vi "Upgrade to Secure Client VISA Socket.vi"(6 "server certificate validation":enum32{"Any Trusted CA", "None"}(ring), 7 "immutable TLS Configuration":refnum<k36>, 8 "error in (no error)":errorcluster, 9 "timeout (5000ms)":i32=5000, 10 "Server Hostname":string, 11 "VISA TCP Socket in":refnum<class "VISA TCP.lvclass">) -> (0 "error out":errorcluster, 2 "server certificate chain":cluster{"certificate":u8[]}[](array[cluster]), 3 "Secure VISA TCP Socket out":refnum<class "VISA TCP.lvclass">)   [LabVIEW 2020, in "Secure Sockets Addon.lvlib"]
doc: "Upgrades a Client VISA TCP socket to use SSL/TLS."
uses:
  <vilib>/MediaMongrels Ltd/WebSockets/Sockets/VISA TCP Socket/VISA TCP.lvclass
  <vilib>/MediaMongrels Ltd/WebSockets/Sockets/VISA TCP Socket/VISA TCP.lvclass/VISA TCP.ctl
  <vilib>/MediaMongrels Ltd/WebSockets/Sockets/VISA TCP Socket/Read TCP Refnum.vi
  <vilib>/MediaMongrels Ltd/WebSockets/Sockets/VISA TCP Socket/Write TCP Refnum.vi
  Secure Sockets Addon.lvlib
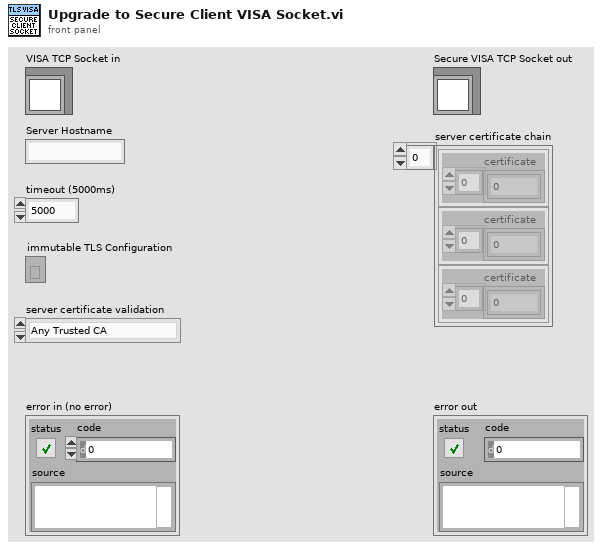
[diagram p1: front panel]
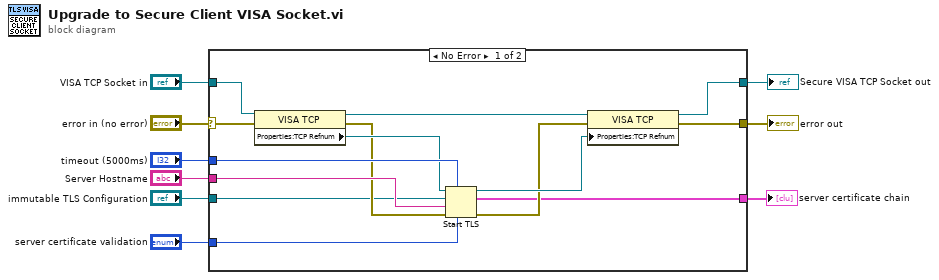
[diagram p0: block diagram]
diagram:
  n1 = case shown="No Error" "error in (no error)" {
    selector: "error in (no error)" -> [w13 w25]
    tunnel: "VISA TCP Socket in" -> [w23 w24]
    tunnel: "Server Hostname" -> [w22 _]
    tunnel: "timeout (5000ms)" -> [w21 _]
    tunnel: [w15 w25] -> w6
    tunnel: [w14 w24] -> w5
    tunnel: "server certificate validation" -> [w12 _]
    tunnel: "immutable TLS Configuration" -> [w11 _]
    tunnel: [w10 _] -> w1
    frame No Error {
      n2 = property class="VISA TCP"(reference=w23, error in=w13) -> (reference out=w18:refnum<class "VISA TCP.lvclass">, error out=w17:errorcluster, "Properties:TCP Refnum"=w20:refnum<k5>)
      n3 = Start TLS(6:w12, 7:w21, 8:w17, 9:w22, 10:w11, 11:w20) -> (0:w16:errorcluster, 2:w10:cluster{"certificate":u8[]}[], 3:w19:refnum<k5>)
      n4 = property class="VISA TCP"(reference=w18, error in=w16, "Properties:TCP Refnum"=w19) -> (reference out=w14:refnum<class "VISA TCP.lvclass">, error out=w15:errorcluster)
    }
    frame Error {
    }
  }
  "error out" <- w6
  "Secure VISA TCP Socket out" <- w5
  "server certificate chain" <- w1
